vi "Wolna_ogranicz_ramke.vi"(6 "size(16000)":i32=16000, 8 "error in (no error)":errorcluster, 9 "Bufor in":T1) -> (0 "error out":errorcluster, 1 "Bufor out":T1)   [LabVIEW 2014]
doc: "Ogranicza długość ramki do rozmiaru size\ndla przebiegów analogowych"
uses:
  Kontrolki/Przetwarzanie/Kanaly.ctl
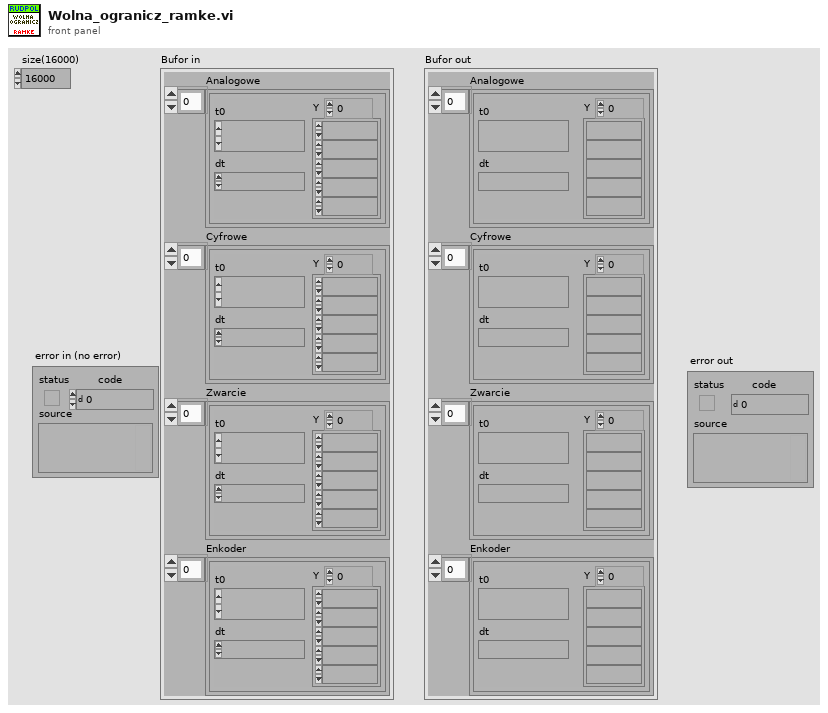
[diagram p1: front panel]
types:
  T1 = typedef "Kanaly.ctl" = cluster{"Analogowe":waveform(dbl)[], "Cyfrowe":waveform(dbl)[], "Zwarcie":waveform(dbl)[], "Enkoder":waveform(dbl)[]}
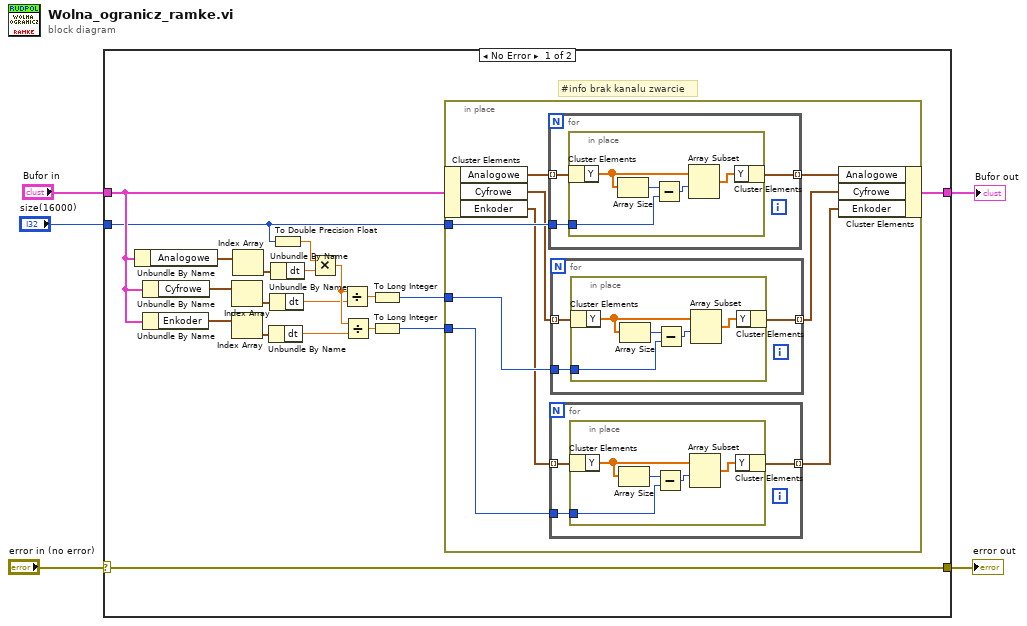
[diagram p0: block diagram]
diagram:
  n1 = case shown="No Error" "error in (no error)" {
    selector: "error in (no error)" -> [w23 w59]
    tunnel: [w23 w59] -> w4
    tunnel: "Bufor in" -> [w19 w58]
    tunnel: "size(16000)" -> [w13 _]
    tunnel: [w24 w58] -> w1
    frame No Error {
      # "#info brak kanalu zwarcie"
      n2 = Unbundle By Name(w19) -> ("Analogowe"=w22:waveform(dbl)[])
      n3 = Unbundle By Name(w19) -> ("Cyfrowe"=w21:waveform(dbl)[])
      n4 = Unbundle By Name(w19) -> ("Enkoder"=w20:waveform(dbl)[])
      n5 = Index Array(array=w21) -> (element=w17:waveform(dbl))  [unwired: 1 in]
      n6 = Index Array(array=w20) -> (element=w16:waveform(dbl))  [unwired: 1 in]
      n7 = Index Array(array=w22) -> (element=w18:waveform(dbl))  [unwired: 1 in]
      n8 = Unbundle By Name(w16) -> ("dt"=w10:dbl)
      n9 = Unbundle By Name(w17) -> ("dt"=w11:dbl)
      n10 = Unbundle By Name(w18) -> ("dt"=w15:dbl)
      n11 = To Double Precision Float(number=w13) -> (double precision float=w14:dbl)
      n12 = Multiply(x=w14, y=w15) -> (x*y=w12:dbl)
      n13 = Divide(x=w12, y=w11) -> (x/y=w9:dbl)
      n14 = Divide(x=w12, y=w10) -> (x/y=w8:dbl)
      n15 = To Long Integer(number=w9) -> (32bit integer=w7:i32)
      n16 = To Long Integer(number=w8) -> (32bit integer=w6:i32)
      n17 = in-place {
        in-place-border: w13 -> [w32]
        in-place-border: w7 -> [w29]
        in-place-border: w6 -> [w25]
        n18 = in-place-cluster #1(w19) -> ("Analogowe"=w33:waveform(dbl)[], "Cyfrowe"=w30:waveform(dbl)[], "Enkoder"=w27:waveform(dbl)[])
        n19 = for {
          tunnel: w33 -> [w52] mode=indexing
          tunnel: w32 -> [w51]
          tunnel: [w50] -> w31 mode=indexing
          n20 = in-place {
            in-place-border: w51 -> [w53]
            n21 = in-place-cluster #2(w52) -> ("Y"=w54:dbl[])
            n22 = Array Size(array=w54) -> (size(s)=w56:i32)
            n23 = Subtract(x=w56, y=w53) -> (x-y=w57:i32)
            n24 = Array Subset(array=w54, index=w57) -> (w55:dbl[])  [unwired: 1 in]
            n25 = in-place-cluster #2("Y"=w55) -> (w50:waveform(dbl))
          }
        }
        n26 = for {
          tunnel: w27 -> [w36] mode=indexing
          tunnel: w25 -> [w35]
          tunnel: [w34] -> w26 mode=indexing
          n27 = in-place {
            in-place-border: w35 -> [w37]
            n28 = in-place-cluster #3(w36) -> ("Y"=w38:dbl[])
            n29 = Array Size(array=w38) -> (size(s)=w40:i32)
            n30 = Subtract(x=w40, y=w37) -> (x-y=w41:i32)
            n31 = Array Subset(array=w38, index=w41) -> (w39:dbl[])  [unwired: 1 in]
            n32 = in-place-cluster #3("Y"=w39) -> (w34:waveform(dbl))
          }
        }
        n33 = for {
          tunnel: w30 -> [w44] mode=indexing
          tunnel: w29 -> [w43]
          tunnel: [w42] -> w28 mode=indexing
          n34 = in-place {
            in-place-border: w43 -> [w45]
            n35 = in-place-cluster #4(w44) -> ("Y"=w46:dbl[])
            n36 = Array Size(array=w46) -> (size(s)=w48:i32)
            n37 = Subtract(x=w48, y=w45) -> (x-y=w49:i32)
            n38 = Array Subset(array=w46, index=w49) -> (w47:dbl[])  [unwired: 1 in]
            n39 = in-place-cluster #4("Y"=w47) -> (w42:waveform(dbl))
          }
        }
        n40 = in-place-cluster #1("Analogowe"=w31, "Cyfrowe"=w28, "Enkoder"=w26) -> (w24:T1)
      }
    }
    frame Error {
    }
  }
  "error out" <- w4
  "Bufor out" <- w1
